vi "_WriteTopData_TDMS_Virtual_CI.vi"(8 "error in (no error)":errorcluster, 10 "Top Data in":T1={"Status"={"id_sensor"=0, "Ind."=FALSE, "sample time"=0, "rov_states"=enum."INIT", "acquisition_time"=timestamp(0 s since 1904-01-01), "modo_ctrl"=enum."Manual"}, "DAQ"={"id_daq"=0, "id_sensor"=0, "gps_"={"lat"=0.0, "lon"=0.0, "alt"=0.0}, "usbl_"={"x"=0.0, "y"=0.0, "z"=0.0}, "vess_ahrs_"={"pitch"=0.0, "roll"=0.0, "yaw"=0.0}, "acquisition_time"=timestamp(0 s since 1904-01-01)}, "User Data"={"id_sensor"=0, "id_daq"=0, "ci_habilitada"=FALSE, "acquisition_time"=timestamp(0 s since 1904-01-01), "CI Data"={"joy_1x"=0.0, "joy_1y"=0.0, "joy_1z"=0.0, "joy_1thumb"=0.0, "joy_1botIzq"=0, "joy_1botder"=0, "joy_1gatillo"=0, "modo_1bot"=0, "modo_2bot"=0, "modo_3bot"=0, "modo_4bot"=0, "pot"=0.0, "enc"=0.0, "joy_2x"=0.0, "joy_2y"=0.0, "joy_2z"=0.0, "joy_2bot"=0, "botella_1bot"=0, "botella_2bot"=0, "botella_3bot"=0, "botella_4bot"=0, "corer_1bot"=0, "corer_2bot"=0, "a_in"=0.0, "dio1"=0, "dio2"=0, "dio3"=0, "ci_acc_x"=0.0, "ci_acc_y"=0.0, "ci_acc_z"=0.0}, "Surface Data"={"modo_1ind"=0, "modo_2ind"=0, "modo_3ind"=0, "modo_4ind"=0, "botella_1ind"=0, "botella_2ind"=0, "botella_3ind"=0, "botella_4ind"=0, "corer_1ind"=0, "corer_2ind"=0, "lars_vel"=0.0, "lars_fwd"=0, "lars_rev"=0}}, "Virtual CI"={"id_sensor"=0, "id_daq"=0, "bus_260v"=FALSE, "m_6"=FALSE, "m_5"=FALSE, "m_2"=FALSE, "m_1"=FALSE, "m_4"=FALSE, "m_3"=FALSE, "luz_1"=FALSE, "luz_2"=FALSE, "luz_3"=FALSE, "pot_m1"=0.0, "pot_m2"=0.0, "pot_m3"=0.0, "pot_m4"=0.0, "pot_m5"=0.0, "pot_m6"=0.0, "pot_l1"=0.0, "pot_l2"=0.0, "pot_l3"=0.0, "pot_gen"=0.0, "fuente_muestras"=FALSE, "bot_1"=FALSE, "bot_2"=FALSE, "bot_3"=FALSE, "bot_4"=FALSE, "corer_1"=FALSE, "corer_2"=FALSE, "pot_c1"=0.0, "pot_c2"=0.0, "virtual_ci"=FALSE, "acquisition_time"=timestamp(0 s since 1904-01-01)}, "Control"={"depth_PID"={"Kp"=0.0, "Ti"=0.03, "Td"=0.001}, "heading_PID"={"Kp"=0.05, "Ti"=0.03, "Td"=0.001}, "altitude_PID"={"Kp"=0.05, "Ti"=0.03, "Td"=0.001}, "depth_sp"=0.0, "heading_sp"=0.0, "altitude_sp"=0.0, "m_PID_en"=FALSE, "PID_reset"=FALSE, "acquisition_time"=timestamp(0 s since 1904-01-01), "motor_PID"={"Kp"=0.05, "Ti"=0.03, "Td"=0.001}, "m1_lo"=0.0, "m1_hi"=0.0, "m1_en"=TRUE, "m2_lo"=0.0, "m2_hi"=0.0, "m2_en"=TRUE, "m3_lo"=0.0, "m3_hi"=0.0, "m3_en"=TRUE, "m4_lo"=0.0, "m4_hi"=5.0, "m4_en"=TRUE, "m5_lo"=-5.0, "m5_hi"=5.0, "m5_en"=TRUE, "m6_lo"=-5.0, "m6_hi"=5.0, "m6_en"=TRUE, "modo_ctrl"=enum."Manual"}} {"Virtual CI"."pot_c2" step=0.1; "Virtual CI"."pot_c1" step=0.01; "Virtual CI"."pot_gen" step=1.0; "Virtual CI"."pot_l3" step=0.01; "Virtual CI"."pot_l2" step=0.01; "Virtual CI"."pot_l1" step=0.01; "Virtual CI"."pot_m6" step=0.01; "Virtual CI"."pot_m5" step=0.01; "Virtual CI"."pot_m4" step=0.01; "Virtual CI"."pot_m3" step=0.01; "Virtual CI"."pot_m2" step=0.01; "Virtual CI"."pot_m1" step=0.01; "DAQ"."vess_ahrs_"."yaw" format="%.2g"; "DAQ"."vess_ahrs_"."roll" format="%.2g"; "DAQ"."vess_ahrs_"."pitch" format="%.2g"; "DAQ"."usbl_"."z" format="%.7g"; "DAQ"."usbl_"."y" format="%.7g"; "DAQ"."usbl_"."x" format="%.7g"; "DAQ"."gps_"."alt" format="%.7g"; "DAQ"."gps_"."lon" format="%.7g"; "DAQ"."gps_"."lat" format="%.7g"}, 11 "Refnum in":refnum<k34>) -> (0 "error out":errorcluster, 3 "Refnum out":refnum<k34>)   [LabVIEW 2018]
uses:
  TypeDefsTopside/Top Data.ctl
  Shared/Type Defs/ROV States.ctl
  TypeDefsSubsea/Modos Control.ctl
  TypeDefsTopside/DAQ Top Data.ctl
  TypeDefsTopside/User Data.ctl
  TypeDefsTopside/CI Data.ctl
  TypeDefsTopside/Surface Input Data.ctl
  TypeDefsTopside/Virtual User Interface Data.ctl
  TypeDefsTopside/Top Control.ctl
  TypeDefsSubsea/Type Defs Subsea.lvlib
  TypeDefsTopside/Type Defs Topside.lvlib
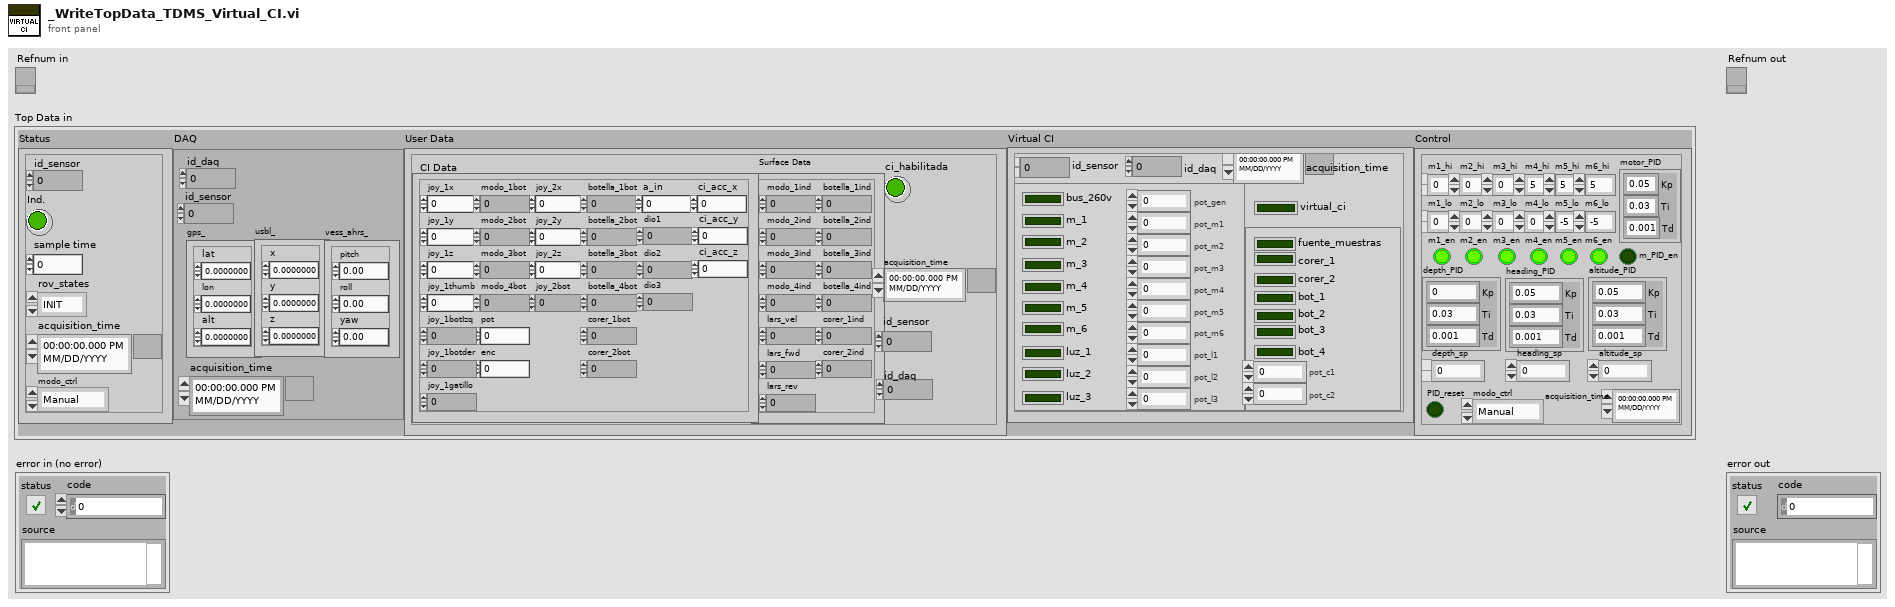
[diagram p1: front panel]
types:
  T1 = typedef "Type Defs Topside.lvlib/Top Data.ctl" = cluster{"Status":cluster{"id_sensor":u32, "Ind.":bool, "sample time":u32, "rov_states":T2, "acquisition_time":timestamp, "modo_ctrl":T3}, "DAQ":T4, "User Data":T5, "Virtual CI":T8, "Control":T9}
  T2 = typedef "Type Defs Subsea.lvlib/ROV States.ctl" = enum16{"INIT", "IDLE", "TEST", "RUN", "EMERGENCY", "EXIT"}
  T3 = typedef "Type Defs Subsea.lvlib/Modos Control.ctl" = enum16{"Manual", "Profundidad", "Altitud", "Rumbo", "P+R"}
  T4 = typedef "Type Defs Topside.lvlib/DAQ Top Data.ctl" = cluster{"id_daq":u32, "id_sensor":u32, "gps_":cluster{"lat":dbl, "lon":dbl, "alt":dbl}, "usbl_":cluster{"x":dbl, "y":dbl, "z":dbl}, "vess_ahrs_":cluster{"pitch":dbl, "roll":dbl, "yaw":dbl}, "acquisition_time":timestamp}
  T5 = typedef "Type Defs Topside.lvlib/User Data.ctl" = cluster{"id_sensor":u32, "id_daq":u64, "ci_habilitada":bool, "acquisition_time":timestamp, "CI Data":T6, "Surface Data":T7}
  T6 = typedef "Type Defs Topside.lvlib/CI Data.ctl" = cluster{"joy_1x":dbl, "joy_1y":dbl, "joy_1z":dbl, "joy_1thumb":dbl, "joy_1botIzq":u8, "joy_1botder":u8, "joy_1gatillo":u8, "modo_1bot":u8, "modo_2bot":u8, "modo_3bot":u8, "modo_4bot":u8, "pot":dbl, "enc":dbl, "joy_2x":dbl, "joy_2y":dbl, "joy_2z":dbl, "joy_2bot":u8, "botella_1bot":u8, "botella_2bot":u8, "botella_3bot":u8, "botella_4bot":u8, "corer_1bot":u8, "corer_2bot":u8, "a_in":dbl, "dio1":u8, "dio2":u8, "dio3":u8, "ci_acc_x":dbl, "ci_acc_y":dbl, "ci_acc_z":dbl}
  T7 = typedef "Type Defs Topside.lvlib/Surface Input Data.ctl" = cluster{"modo_1ind":u8, "modo_2ind":u8, "modo_3ind":u8, "modo_4ind":u8, "botella_1ind":u8, "botella_2ind":u8, "botella_3ind":u8, "botella_4ind":u8, "corer_1ind":u8, "corer_2ind":u8, "lars_vel":dbl, "lars_fwd":u8, "lars_rev":u8}
  T8 = typedef "Type Defs Topside.lvlib/Virtual User Interface Data.ctl" = cluster{"id_sensor":u32, "id_daq":u64, "bus_260v":bool, "m_6":bool, "m_5":bool, "m_2":bool, "m_1":bool, "m_4":bool, "m_3":bool, "luz_1":bool, "luz_2":bool, "luz_3":bool, "pot_m1":dbl, "pot_m2":dbl, "pot_m3":dbl, "pot_m4":dbl, "pot_m5":dbl, "pot_m6":dbl, "pot_l1":dbl, "pot_l2":dbl, "pot_l3":dbl, "pot_gen":dbl, "fuente_muestras":bool, "bot_1":bool, "bot_2":bool, "bot_3":bool, "bot_4":bool, "corer_1":bool, "corer_2":bool, "pot_c1":dbl, "pot_c2":dbl, "virtual_ci":bool, "acquisition_time":timestamp}
  T9 = typedef "Type Defs Topside.lvlib/Top Control.ctl" = cluster{"depth_PID":cluster{"Kp":dbl, "Ti":dbl, "Td":dbl}, "heading_PID":cluster{"Kp":dbl, "Ti":dbl, "Td":dbl}, "altitude_PID":cluster{"Kp":dbl, "Ti":dbl, "Td":dbl}, "depth_sp":dbl, "heading_sp":dbl, "altitude_sp":dbl, "m_PID_en":bool, "PID_reset":bool, "acquisition_time":timestamp, "motor_PID":cluster{"Kp":dbl, "Ti":dbl, "Td":dbl}, "m1_lo":dbl, "m1_hi":dbl, "m1_en":bool, "m2_lo":dbl, "m2_hi":dbl, "m2_en":bool, "m3_lo":dbl, "m3_hi":dbl, "m3_en":bool, "m4_lo":dbl, "m4_hi":dbl, "m4_en":bool, "m5_lo":dbl, "m5_hi":dbl, "m5_en":bool, "m6_lo":dbl, "m6_hi":dbl, "m6_en":bool, "modo_ctrl":T3}
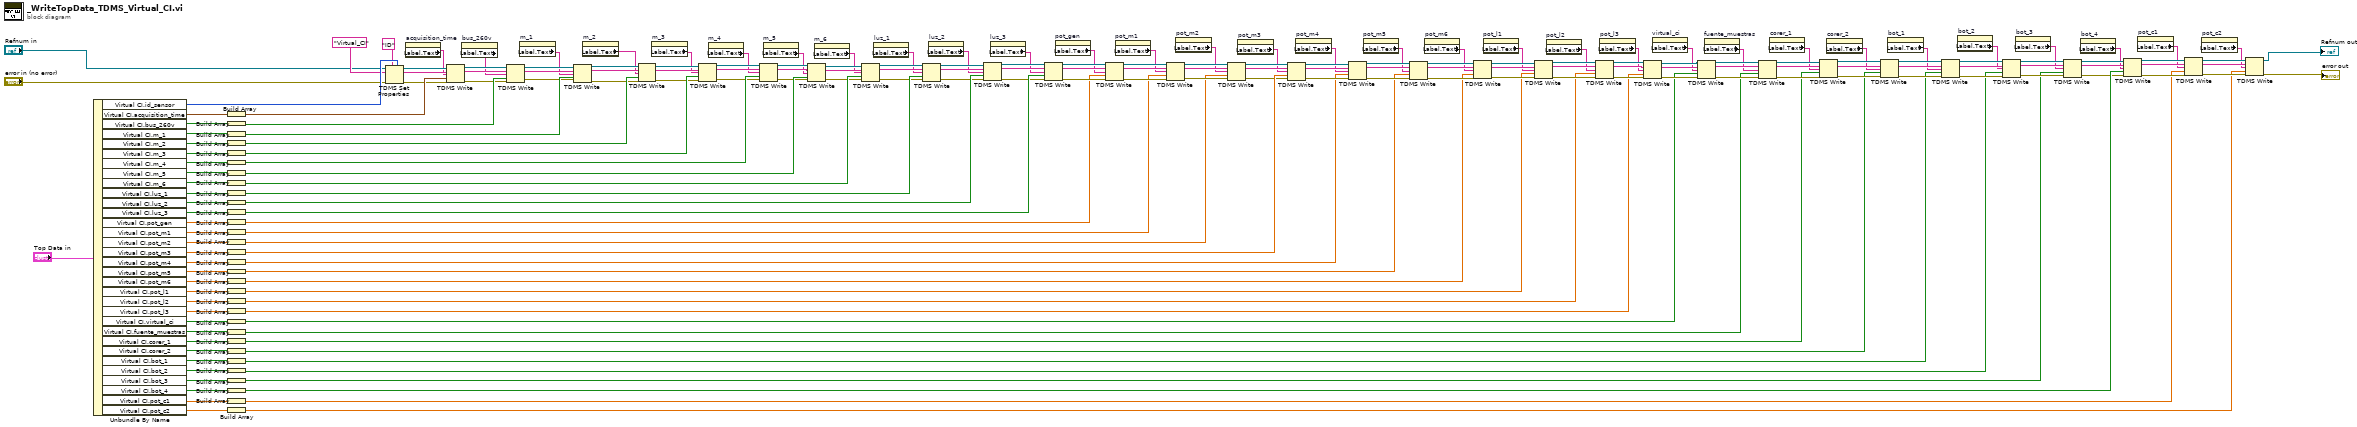
[diagram p0: block diagram]
diagram:
  n1 = Unbundle By Name("Top Data in") -> ("Virtual CI.id_sensor"=w183:u32, "Virtual CI.acquisition_time"=w64:timestamp, "Virtual CI.bus_260v"=w63:bool, "Virtual CI.m_1"=w62:bool, "Virtual CI.m_2"=w61:bool, "Virtual CI.m_3"=w60:bool, "Virtual CI.m_4"=w59:bool, "Virtual CI.m_5"=w58:bool, "Virtual CI.m_6"=w57:bool, "Virtual CI.luz_1"=w56:bool, "Virtual CI.luz_2"=w55:bool, "Virtual CI.luz_3"=w54:bool, "Virtual CI.pot_gen"=w53:dbl, "Virtual CI.pot_m1"=w52:dbl, "Virtual CI.pot_m2"=w51:dbl, "Virtual CI.pot_m3"=w50:dbl, "Virtual CI.pot_m4"=w49:dbl, "Virtual CI.pot_m5"=w48:dbl, "Virtual CI.pot_m6"=w47:dbl, "Virtual CI.pot_l1"=w46:dbl, "Virtual CI.pot_l2"=w45:dbl, "Virtual CI.pot_l3"=w44:dbl, "Virtual CI.virtual_ci"=w43:bool, "Virtual CI.fuente_muestras"=w42:bool, "Virtual CI.corer_1"=w21:bool, "Virtual CI.corer_2"=w22:bool, "Virtual CI.bot_1"=w23:bool, "Virtual CI.bot_2"=w24:bool, "Virtual CI.bot_3"=w25:bool, "Virtual CI.bot_4"=w26:bool, "Virtual CI.pot_c1"=w27:dbl, "Virtual CI.pot_c2"=w28:dbl)
  n2 = Build Array(w64) -> (w184:timestamp[])
  n3 = Build Array(w63) -> (w185:bool[])
  n4 = Build Array(w62) -> (w186:bool[])
  n5 = Build Array(w61) -> (w187:bool[])
  n6 = Build Array(w60) -> (w188:bool[])
  n7 = Build Array(w59) -> (w189:bool[])
  n8 = Build Array(w58) -> (w190:bool[])
  n9 = Build Array(w57) -> (w191:bool[])
  n10 = Build Array(w56) -> (w192:bool[])
  n11 = Build Array(w55) -> (w193:bool[])
  n12 = Build Array(w54) -> (w194:bool[])
  n13 = Build Array(w53) -> (w145:dbl[])
  n14 = Build Array(w52) -> (w144:dbl[])
  n15 = Build Array(w51) -> (w143:dbl[])
  n16 = Build Array(w50) -> (w92:dbl[])
  n17 = Build Array(w49) -> (w91:dbl[])
  n18 = Build Array(w48) -> (w90:dbl[])
  n19 = Build Array(w47) -> (w89:dbl[])
  n20 = Build Array(w46) -> (w88:dbl[])
  n21 = Build Array(w45) -> (w87:dbl[])
  n22 = Build Array(w44) -> (w86:dbl[])
  n23 = Build Array(w43) -> (w85:bool[])
  n24 = Build Array(w42) -> (w84:bool[])
  n25 = Build Array(w21) -> (w83:bool[])
  n26 = Build Array(w22) -> (w82:bool[])
  n27 = Build Array(w23) -> (w81:bool[])
  n28 = Build Array(w24) -> (w80:bool[])
  n29 = Build Array(w25) -> (w79:bool[])
  n30 = Build Array(w26) -> (w78:bool[])
  n31 = Build Array(w27) -> (w77:dbl[])
  n32 = Build Array(w28) -> (w76:dbl[])
  n33 = TDMS Set Properties(5:w183, 7:"ID" ("property names"), 8:"error in (no error)", 10:"Virtual_CI" ("group name in (Untitled)"), 11:"Refnum in") -> (0:w161:errorcluster, 2:w160:string, 3:w158:refnum<k34>)  [unwired: 1 in, 1 out]
  n34 = property on="acquisition_time" class="AbsTime (strict)"() -> ("Label.Text"=w38:string)  [unwired: 2 in, 2 out]
  n35 = TDMS Write(0:w158, 5:w160, 7:w38, 9:w184, 11:w161) -> (4:w156:refnum<k34>, 6:w155:string, 15:w157:errorcluster)  [unwired: 1 in, 1 out]
  n36 = property on="bus_260v" class="Bool (strict)"() -> ("Label.Text"=w39:string)  [unwired: 2 in, 2 out]
  n37 = TDMS Write(0:w156, 5:w155, 7:w39, 9:w185, 11:w157) -> (4:w67:refnum<k34>, 6:w66:string, 15:w65:errorcluster)  [unwired: 1 in, 1 out]
  n38 = property on="m_1" class="Bool (strict)"() -> ("Label.Text"=w37:string)  [unwired: 2 in, 2 out]
  n39 = TDMS Write(0:w67, 5:w66, 7:w37, 9:w186, 11:w65) -> (4:w141:refnum<k34>, 6:w140:string, 15:w142:errorcluster)  [unwired: 1 in, 1 out]
  n40 = property on="m_2" class="Bool (strict)"() -> ("Label.Text"=w36:string)  [unwired: 2 in, 2 out]
  n41 = TDMS Write(0:w141, 5:w140, 7:w36, 9:w187, 11:w142) -> (4:w163:refnum<k34>, 6:w164:string, 15:w162:errorcluster)  [unwired: 1 in, 1 out]
  n42 = property on="m_3" class="Bool (strict)"() -> ("Label.Text"=w35:string)  [unwired: 2 in, 2 out]
  n43 = TDMS Write(0:w163, 5:w164, 7:w35, 9:w188, 11:w162) -> (4:w166:refnum<k34>, 6:w167:string, 15:w165:errorcluster)  [unwired: 1 in, 1 out]
  n44 = property on="m_4" class="Bool (strict)"() -> ("Label.Text"=w34:string)  [unwired: 2 in, 2 out]
  n45 = TDMS Write(0:w166, 5:w167, 7:w34, 9:w189, 11:w165) -> (4:w179:refnum<k34>, 6:w181:string, 15:w180:errorcluster)  [unwired: 1 in, 1 out]
  n46 = property on="m_5" class="Bool (strict)"() -> ("Label.Text"=w33:string)  [unwired: 2 in, 2 out]
  n47 = TDMS Write(0:w179, 5:w181, 7:w33, 9:w190, 11:w180) -> (4:w177:refnum<k34>, 6:w178:string, 15:w182:errorcluster)  [unwired: 1 in, 1 out]
  n48 = property on="m_6" class="Bool (strict)"() -> ("Label.Text"=w32:string)  [unwired: 2 in, 2 out]
  n49 = TDMS Write(0:w177, 5:w178, 7:w32, 9:w191, 11:w182) -> (4:w175:refnum<k34>, 6:w176:string, 15:w174:errorcluster)  [unwired: 1 in, 1 out]
  n50 = property on="luz_1" class="Bool (strict)"() -> ("Label.Text"=w31:string)  [unwired: 2 in, 2 out]
  n51 = TDMS Write(0:w175, 5:w176, 7:w31, 9:w192, 11:w174) -> (4:w169:refnum<k34>, 6:w170:string, 15:w168:errorcluster)  [unwired: 1 in, 1 out]
  n52 = property on="luz_2" class="Bool (strict)"() -> ("Label.Text"=w30:string)  [unwired: 2 in, 2 out]
  n53 = TDMS Write(0:w169, 5:w170, 7:w30, 9:w193, 11:w168) -> (4:w172:refnum<k34>, 6:w173:string, 15:w171:errorcluster)  [unwired: 1 in, 1 out]
  n54 = property on="luz_3" class="Bool (strict)"() -> ("Label.Text"=w29:string)  [unwired: 2 in, 2 out]
  n55 = TDMS Write(0:w172, 5:w173, 7:w29, 9:w194, 11:w171) -> (4:w147:refnum<k34>, 6:w139:string, 15:w146:errorcluster)  [unwired: 1 in, 1 out]
  n56 = property on="pot_gen" class="DigNum (strict)"() -> ("Label.Text"=w20:string)  [unwired: 2 in, 2 out]
  n57 = TDMS Write(0:w147, 5:w139, 7:w20, 9:w145, 11:w146) -> (4:w149:refnum<k34>, 6:w150:string, 15:w148:errorcluster)  [unwired: 1 in, 1 out]
  n58 = property on="pot_m1" class="DigNum (strict)"() -> ("Label.Text"=w19:string)  [unwired: 2 in, 2 out]
  n59 = TDMS Write(0:w149, 5:w150, 7:w19, 9:w144, 11:w148) -> (4:w152:refnum<k34>, 6:w153:string, 15:w151:errorcluster)  [unwired: 1 in, 1 out]
  n60 = property on="pot_m2" class="DigNum (strict)"() -> ("Label.Text"=w18:string)  [unwired: 2 in, 2 out]
  n61 = TDMS Write(0:w152, 5:w153, 7:w18, 9:w143, 11:w151) -> (4:w71:refnum<k34>, 6:w69:string, 15:w70:errorcluster)  [unwired: 1 in, 1 out]
  n62 = property on="pot_m3" class="DigNum (strict)"() -> ("Label.Text"=w17:string)  [unwired: 2 in, 2 out]
  n63 = TDMS Write(0:w71, 5:w69, 7:w17, 9:w92, 11:w70) -> (4:w115:refnum<k34>, 6:w114:string, 15:w116:errorcluster)  [unwired: 1 in, 1 out]
  n64 = property on="pot_m4" class="DigNum (strict)"() -> ("Label.Text"=w16:string)  [unwired: 2 in, 2 out]
  n65 = TDMS Write(0:w115, 5:w114, 7:w16, 9:w91, 11:w116) -> (4:w112:refnum<k34>, 6:w111:string, 15:w113:errorcluster)  [unwired: 1 in, 1 out]
  n66 = property on="pot_m5" class="DigNum (strict)"() -> ("Label.Text"=w15:string)  [unwired: 2 in, 2 out]
  n67 = TDMS Write(0:w112, 5:w111, 7:w15, 9:w90, 11:w113) -> (4:w101:refnum<k34>, 6:w100:string, 15:w102:errorcluster)  [unwired: 1 in, 1 out]
  n68 = property on="pot_m6" class="DigNum (strict)"() -> ("Label.Text"=w14:string)  [unwired: 2 in, 2 out]
  n69 = TDMS Write(0:w101, 5:w100, 7:w14, 9:w89, 11:w102) -> (4:w118:refnum<k34>, 6:w119:string, 15:w117:errorcluster)  [unwired: 1 in, 1 out]
  n70 = property on="pot_l1" class="DigNum (strict)"() -> ("Label.Text"=w13:string)  [unwired: 2 in, 2 out]
  n71 = TDMS Write(0:w118, 5:w119, 7:w13, 9:w88, 11:w117) -> (4:w121:refnum<k34>, 6:w122:string, 15:w120:errorcluster)  [unwired: 1 in, 1 out]
  n72 = property on="pot_l2" class="DigNum (strict)"() -> ("Label.Text"=w12:string)  [unwired: 2 in, 2 out]
  n73 = TDMS Write(0:w121, 5:w122, 7:w12, 9:w87, 11:w120) -> (4:w134:refnum<k34>, 6:w136:string, 15:w135:errorcluster)  [unwired: 1 in, 1 out]
  n74 = property on="pot_l3" class="DigNum (strict)"() -> ("Label.Text"=w11:string)  [unwired: 2 in, 2 out]
  n75 = TDMS Write(0:w134, 5:w136, 7:w11, 9:w86, 11:w135) -> (4:w132:refnum<k34>, 6:w133:string, 15:w137:errorcluster)  [unwired: 1 in, 1 out]
  n76 = property on="virtual_ci" class="Bool (strict)"() -> ("Label.Text"=w10:string)  [unwired: 2 in, 2 out]
  n77 = TDMS Write(0:w132, 5:w133, 7:w10, 9:w85, 11:w137) -> (4:w130:refnum<k34>, 6:w131:string, 15:w129:errorcluster)  [unwired: 1 in, 1 out]
  n78 = property on="fuente_muestras" class="Bool (strict)"() -> ("Label.Text"=w9:string)  [unwired: 2 in, 2 out]
  n79 = TDMS Write(0:w130, 5:w131, 7:w9, 9:w84, 11:w129) -> (4:w124:refnum<k34>, 6:w125:string, 15:w123:errorcluster)  [unwired: 1 in, 1 out]
  n80 = property on="corer_1" class="Bool (strict)"() -> ("Label.Text"=w8:string)  [unwired: 2 in, 2 out]
  n81 = TDMS Write(0:w124, 5:w125, 7:w8, 9:w83, 11:w123) -> (4:w127:refnum<k34>, 6:w128:string, 15:w126:errorcluster)  [unwired: 1 in, 1 out]
  n82 = property on="corer_2" class="Bool (strict)"() -> ("Label.Text"=w7:string)  [unwired: 2 in, 2 out]
  n83 = TDMS Write(0:w127, 5:w128, 7:w7, 9:w82, 11:w126) -> (4:w104:refnum<k34>, 6:w99:string, 15:w103:errorcluster)  [unwired: 1 in, 1 out]
  n84 = property on="bot_1" class="Bool (strict)"() -> ("Label.Text"=w6:string)  [unwired: 2 in, 2 out]
  n85 = TDMS Write(0:w104, 5:w99, 7:w6, 9:w81, 11:w103) -> (4:w106:refnum<k34>, 6:w107:string, 15:w105:errorcluster)  [unwired: 1 in, 1 out]
  n86 = property on="bot_2" class="Bool (strict)"() -> ("Label.Text"=w5:string)  [unwired: 2 in, 2 out]
  n87 = TDMS Write(0:w106, 5:w107, 7:w5, 9:w80, 11:w105) -> (4:w109:refnum<k34>, 6:w110:string, 15:w108:errorcluster)  [unwired: 1 in, 1 out]
  n88 = property on="bot_3" class="Bool (strict)"() -> ("Label.Text"=w4:string)  [unwired: 2 in, 2 out]
  n89 = TDMS Write(0:w109, 5:w110, 7:w4, 9:w79, 11:w108) -> (4:w74:refnum<k34>, 6:w68:string, 15:w75:errorcluster)  [unwired: 1 in, 1 out]
  n90 = property on="bot_4" class="Bool (strict)"() -> ("Label.Text"=w3:string)  [unwired: 2 in, 2 out]
  n91 = TDMS Write(0:w74, 5:w68, 7:w3, 9:w78, 11:w75) -> (4:w97:refnum<k34>, 6:w96:string, 15:w98:errorcluster)  [unwired: 1 in, 1 out]
  n92 = property on="pot_c1" class="DigNum (strict)"() -> ("Label.Text"=w2:string)  [unwired: 2 in, 2 out]
  n93 = TDMS Write(0:w97, 5:w96, 7:w2, 9:w77, 11:w98) -> (4:w94:refnum<k34>, 6:w93:string, 15:w95:errorcluster)  [unwired: 1 in, 1 out]
  n94 = property on="pot_c2" class="DigNum (strict)"() -> ("Label.Text"=w1:string)  [unwired: 2 in, 2 out]
  n95 = TDMS Write(0:w94, 5:w93, 7:w1, 9:w76, 11:w95) -> (4:→"Refnum out":refnum<k34>, 15:→"error out":errorcluster)  [unwired: 1 in, 2 out]
